vi "BRig_dataTrial_n_ENL2.vi"() -> (2 "output_ENL2_n":i32)   [LabVIEW 2014]
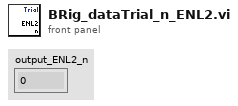
[diagram p1: front panel]
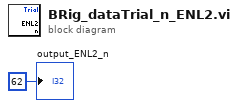
[diagram p0: block diagram]
diagram:
  "output_ENL2_n" <- 62 ("output_iBlock")
